vi "Wait for Acquisition Complete.vi"(8 "error in (no error)":errorcluster, 10 "Maximum Time (10000 ms)":u32=10000, 11 "VISA resource name":refnum<visa-resource-name>) -> (0 "error out":errorcluster, 3 "VISA resource name out":refnum<visa-resource-name>)   [LabVIEW 2010, in "Agilent 3458.lvlib"]
doc: "Waits for a signal from the DMM indicating that requested data is available. This is important especially if there is a lot of data and its important that all of it be retrieved and be outputed. This VI indicates when all of the measurements requested has been retrieved successfully from memory and is now available in the output buffer to be read by VISA.\n\n<B>Note:</B> Use this VI only with other low-level VIs. The high-level VIs automatically incorporate this functionality. This VI does not check the instrument status. If you want to check the instrument status, call the Error Query VI at the conclusion of the sequence."
uses:
  <instrlib>/Agilent 3458/Agilent 3458.lvlib
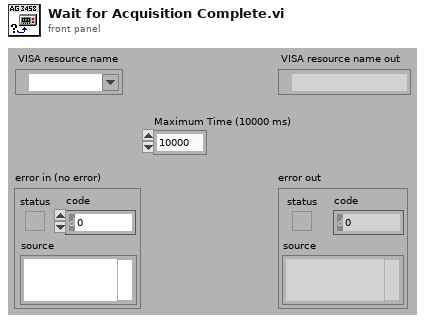
[diagram p1: front panel]
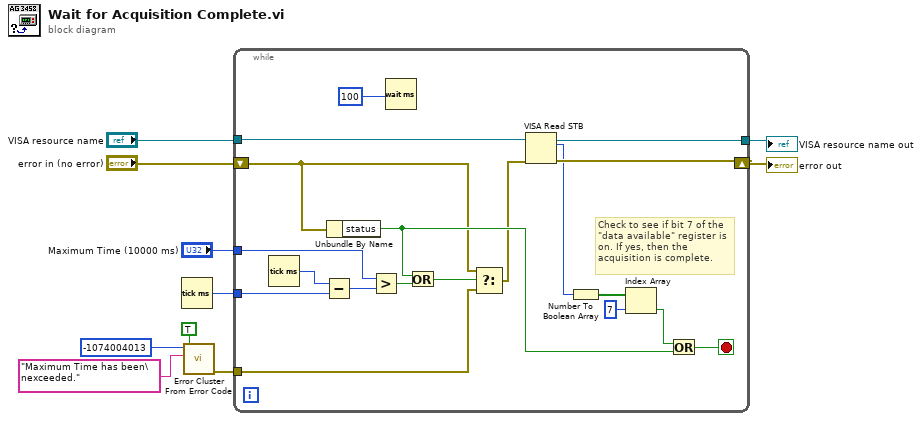
[diagram p0: block diagram]
diagram:
  n1 = Tick Count (ms)() -> (millisecond timer value=w7:u32)
  n2 = call <vilib>:"Error Cluster From Error Code.vi"("show call chain? (False)"=TRUE, "error message (\"\")"="Maximum Time has been\nexceeded." ("error message (\"\")"), "error code (0)"=-1074004013) -> ("error out"=w3:errorcluster)  [unwired: 6 in]
  n3 = while {
    tunnel: "VISA resource name" -> [w18]
    tunnel: "Maximum Time (10000 ms)" -> [w26]
    tunnel: w7 -> [w27]
    tunnel: w3 -> [w23]
    shift-right: [w15] -> w2
    shift-left: "error in (no error)" -> [w19]
    tunnel: [w16] -> w1
    stop <- w22 stop-if-true
    # "Check to see if bit 7 of the \"data available\" register is on. If yes, then the acquisition is complete."
    n4 = Tick Count (ms)() -> (millisecond timer value=w29:u32)
    n5 = Subtract(x=w29, y=w27) -> (x-y=w28:u32)
    n6 = Unbundle By Name(w19) -> ("status"=w21:bool)
    n7 = Greater?(x=w26, y=w28) -> (0:w25:bool)
    n8 = Wait (ms)(milliseconds to wait=u32 100 ("millisecond multiple")) -> ()  [unwired: 1 out]
    n9 = Or(x=w21, y=w25) -> (x .or. y?=w24:bool)
    n10 = Select(t=w19, s=w24, f=w23) -> (s? t:f=w17:errorcluster)
    n11 = VISA Read STB(8:w17, 11:w18) -> (0:w15:errorcluster, 2:w12:u16, 3:w16:refnum<visa-resource-name>)
    n12 = Number To Boolean Array(number=w12) -> (Boolean array=w14:bool[])
    n13 = Index Array(array=w14, index=7) -> (element=w13:bool)
    n14 = Or(x=w13, y=w21) -> (x .or. y?=w22:bool)
  }
  "error out" <- w2
  "VISA resource name out" <- w1
